vi "1.8-Wait on Enum.vi"   [LabVIEW 2010]
uses:
  2-Low Neurons/2.0-Hindbrain Startup State.ctl
  1.0-Hindbrain Global.vi
types:
  T1 = typedef "2.0-Hindbrain Startup State.ctl" = enum8{"Waiting to Run", "Running", "Restart", "Shutdown", "Off"}
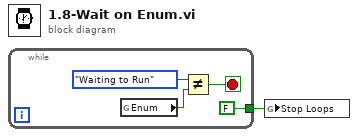
[diagram p0: block diagram]
diagram:
  n1 = while {
    tunnel: [FALSE] -> w1
    stop <- w3 stop-if-true
    n2 = global read "1.0-Hindbrain Global.vi" "Enum"() -> (w5:T1)
    n3 = Not Equal?(x=2.0-Hindbrain_Startup_State."Waiting to Run" ("y"), y=w5) -> (x != y?=w3:bool)
  }
  n4 = global write "1.0-Hindbrain Global.vi" "Stop Loops"(w1) -> ()
